vi "gmmregRegistration.vi"(5 "lambda":dbl[](array[numeric]), 7 "scale":dbl[](array[numeric]), 8 "scene":dbl[][](array[numeric]), 9 "model":dbl[][](array[numeric]), 10 "ctrlPoints":dbl[][](array[numeric]), 11 "param0":dbl[](array[numeric])) -> (0 "denormParams out":dbl[](array[numeric]), 1 "normParams out":dbl[](array[numeric]), 2 "out":dbl[][](array[numeric]), 3 "param0 out":dbl[](array[numeric]) format="%#_8e")   [LabVIEW 2017]
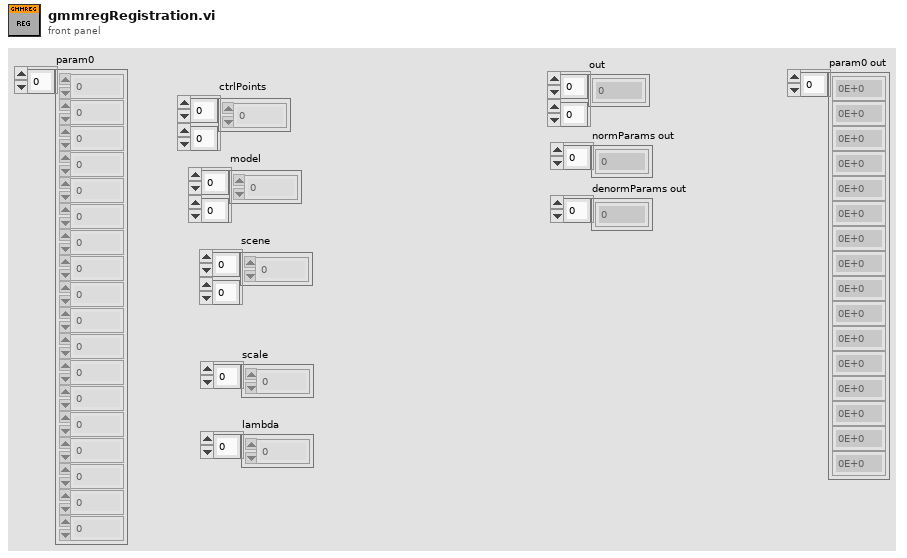
[diagram p1: front panel]
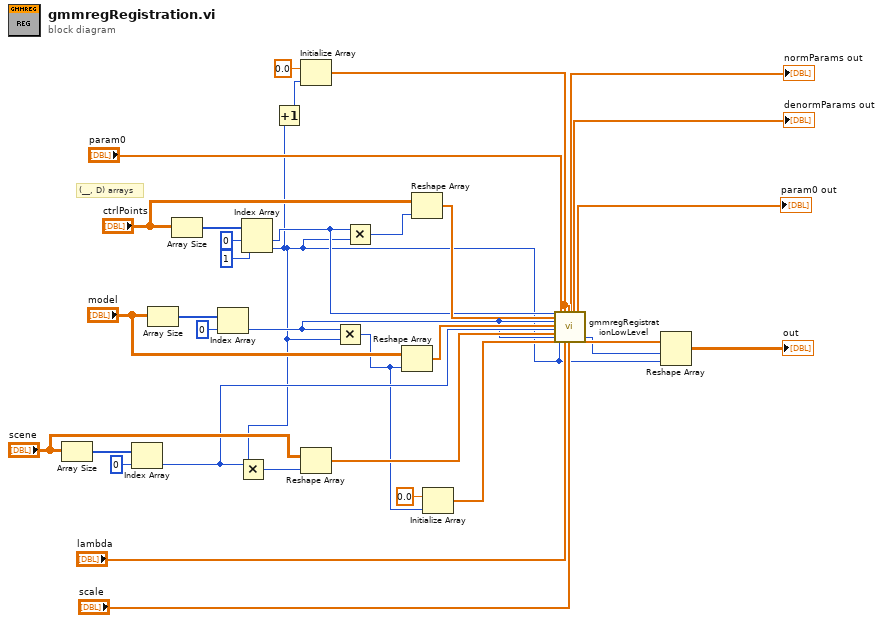
[diagram p0: block diagram]
diagram:
  # "(__, D) arrays"
  n1 = Array Size(array="scene") -> (size(s)=w22:i32[])
  n2 = Index Array(array=w22, index=0) -> (element=w18:i32)
  n3 = Array Size(array="model") -> (size(s)=w34:i32[])
  n4 = Array Size(array="ctrlPoints") -> (size(s)=w31:i32[])
  n5 = Index Array(array=w34, index=0) -> (element=w17:i32)
  n6 = Index Array(array=w31, index #1=0 ("index"), index #2=1 ("index")) -> (element #1=w26:i32, element #2=w6:i32)
  n7 = Multiply(x=w18, y=w6) -> (x*y=w21:i32)
  n8 = Increment(x=w6) -> (x+1=w1:i32)
  n9 = Initialize Array(0.0 ("element"), w1) -> (w4:dbl[])
  n10 = Reshape Array("scene", w21) -> (w19:dbl[])
  n11 = Multiply(x=w17, y=w6) -> (x*y=w16:i32)
  n12 = Multiply(x=w26, y=w6) -> (x*y=w28:i32)
  n13 = Reshape Array("model", w16) -> (w24:dbl[])
  n14 = Reshape Array("ctrlPoints", w28) -> (w27:dbl[])
  n15 = Initialize Array(0.0 ("element"), w16) -> (w14:dbl[])
  n16 = call "gmmregRegistrationLowLevel.vi"("nctrlpts"=w26, "coordCtrlPts"=w27, "npts"=w17, "coord"=w24, "nptsScene"=w18, "coordScene"=w19, "nOut"=w17, "out"=w14, "param0"="param0", "dim (3)"=w6, "normParams"=w4, "lambda"="lambda", "denormParams"=w4, "scale"="scale") -> ("normParams out"=→"normParams out":dbl[], "denormParams out"=→"denormParams out":dbl[], "param0 out"=→"param0 out":dbl[], "nOut out"=w11:i32, "out out"=w12:dbl[])  [unwired: 9 out]
  n17 = Reshape Array(w12, w11, w6) -> (→"out":dbl[][])
